vi "AE - Bluetooth Get Reference.vi"(8 "error in (no error)":errorcluster, 11 "Wiimote":u8) -> (0 "error out":errorcluster, 3 "Wiimote Reference":refnum<k24>)   [LabVIEW 2010]
uses:
  C:/Users/×ñÞóôïò/Desktop/Systems real time/koupe proj/experiments 2/Resources/WiimoteLib.dll
  experiments 2/Resources/WiimoteLib.dll
  AE Cores/AE - Bluetooth Enum.ctl
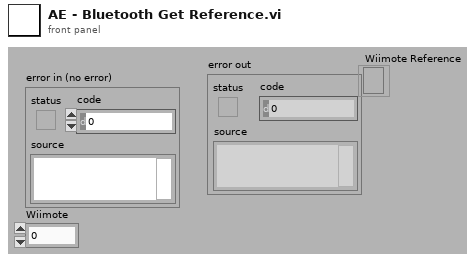
[diagram p1: front panel]
types:
  T1 = typedef "AE - Bluetooth Enum.ctl" = enum16{"Initialise", "Pair All Wiimotes", "Connect All Wiimotes", "Set Rumble", "Set LED", "Get Button + Acc Data", "Get IR Data", "Get Battery", "Get Wiimote Reference", "Reorder Wiimotes", "devReport"}
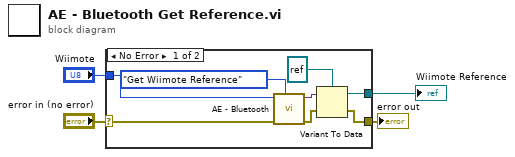
[diagram p0: block diagram]
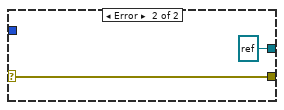
[diagram p2: hidden frame]
diagram:
  n1 = case shown="No Error" "error in (no error)" {
    selector: "error in (no error)" -> [w11 w14]
    tunnel: [w7 w14] -> w3
    tunnel: "Wiimote" -> [w10 _]
    tunnel: [w5 refnum<k24> refnum ("element")] -> w1
    frame No Error {
      n2 = call "AE - Bluetooth.vi"("Enum"=AE_-_Bluetooth_Enum."Get Wiimote Reference", "error in (no error)"=w11, "Variant In"=w10) -> ("error out"=w8:errorcluster, "Variant Out"=w9:variant)  [unwired: 6 in, 1 out]
      n3 = Variant To Data(error in=w8, Variant=w9, type=refnum<k24> refnum ("element")) -> (error out=w7:errorcluster, data=w5:refnum<k24>)
    }
    frame Error {
    }
  }
  "error out" <- w3
  "Wiimote Reference" <- w1
